vi "Wrapper_openAllSpectrometers.vi"(0 "Wrapper In":u32, 1 "error in (no error)":errorcluster) -> (2 "Number of Spectrometers":i32, 3 "Wrapper Out":u32, 4 "error out":errorcluster)   [LabVIEW 2012]
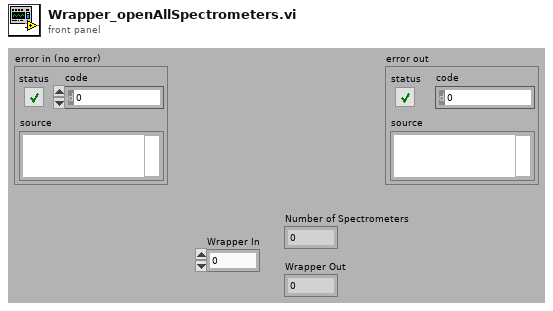
[diagram p1: front panel]
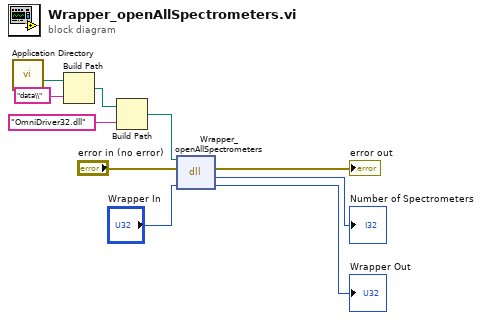
[diagram p0: block diagram]
diagram:
  n1 = call <vilib>:"Application Directory.vi"() -> ("Application Directory"=w7:path)
  n2 = Build Path(base path=w7, name or relative path="data\\") -> (appended path=w4:path)
  n3 = Build Path(base path=w4, name or relative path="OmniDriver32.dll") -> (appended path=w3:path)
  n4 = dll-call lib="D:/Software Development/EPI Development/BurnIn Testing/Instruments/Drivers/Ocean Optics/OOI_HOME/OmniDriver32.dll" fn="Wrapper_openAllSpectrometers" label="Wrapper.openAllSpectrometers"(path in=w3, error in="error in (no error)", "Wrapper"="Wrapper In") -> (error out=→"error out":errorcluster, "return type"=→"Number of Spectrometers":i32, "Wrapper"=→"Wrapper Out":u32)  [unwired: 1 in, 1 out]
